vi "CreateDUTNode.vi"(7 "DOM Document":refnum<k20>, 8 "Error In":errorcluster, 11 "DUT Configuration":T1={"Count"=1, "Wirings"=[], "Names"=[]}) -> (0 "Error Out":errorcluster, 3 "DUT Node":refnum<k20>)   [LabVIEW 2013]
uses:
  DUTConfiguration.ctl
  driver/Public/Controls/SMUSense.ctl
  libs/LV-Utilities/LV-Utilities.lvlib
  driver/Keithley-2602.lvlib
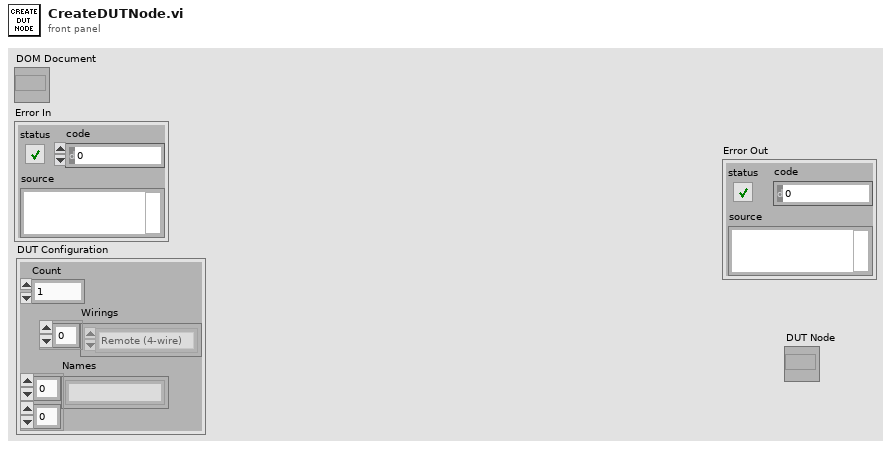
[diagram p1: front panel]
types:
  T1 = typedef "DUTConfiguration.ctl" = cluster{"Count":u32, "Wirings":T2[], "Names":string[][]}
  T2 = typedef "Keithley-2602.lvlib/SMUSense.ctl" = enum16{"Local (2-wire)", "Remote (4-wire)", "Calibration"}
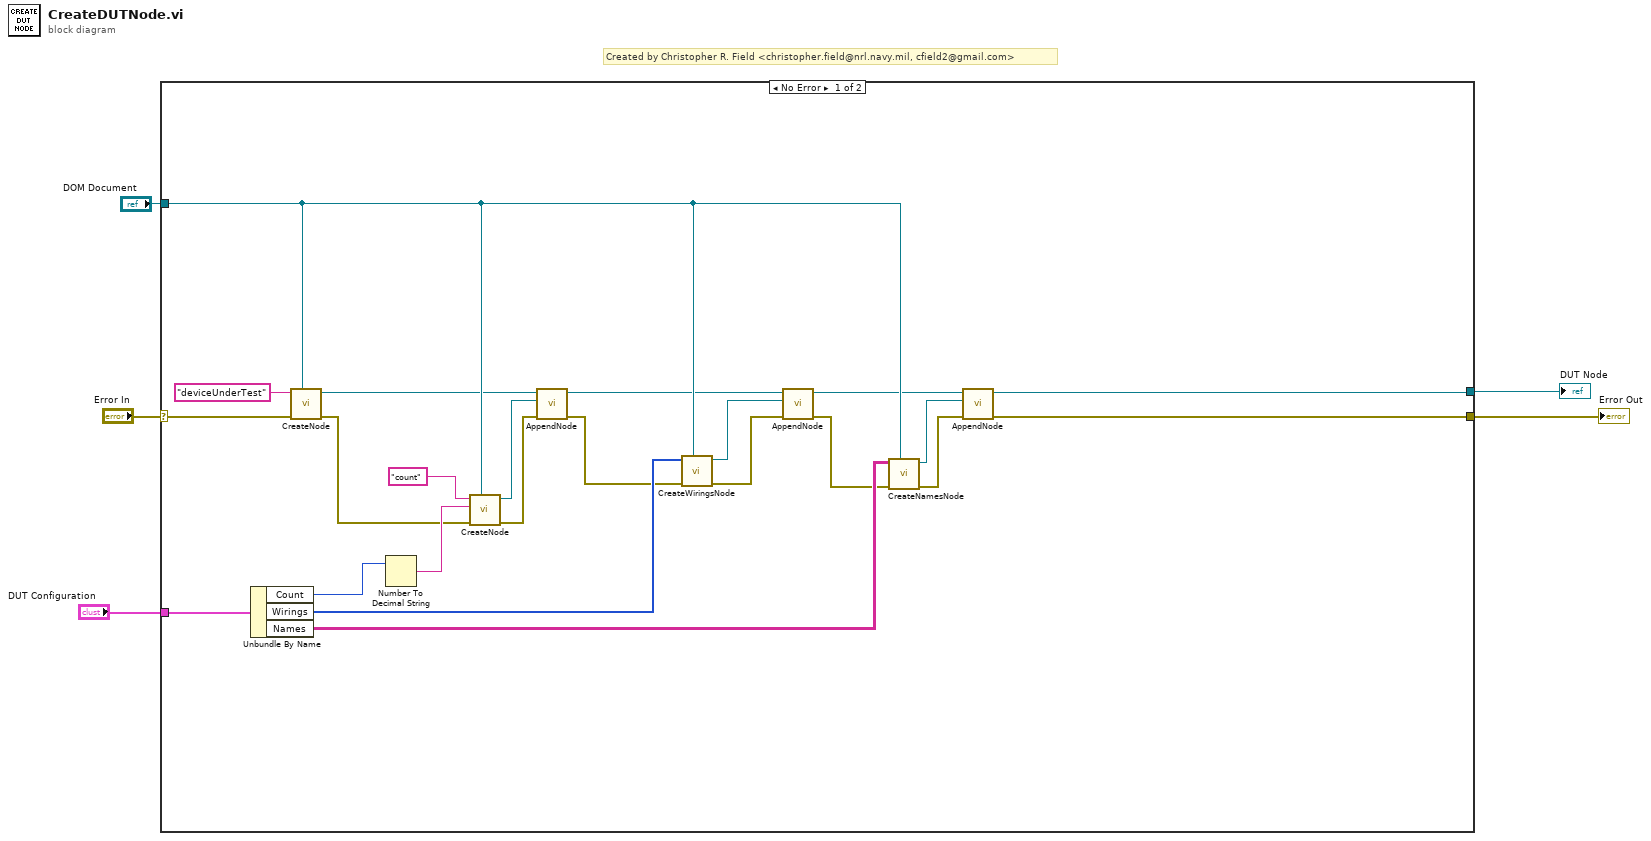
[diagram p0: block diagram]
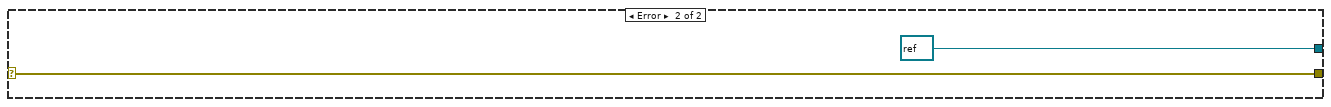
[diagram p2: hidden frame]
diagram:
  # "Created by Christopher R. Field <christopher.field@nrl.navy.mil, cfield2@gmail.com>"
  n1 = case shown="No Error" "Error In" {
    selector: "Error In" -> [w22 w30]
    tunnel: "DOM Document" -> [w20 _]
    tunnel: [w14 w30] -> w3
    tunnel: [w15 refnum<k20> refnum ("DUT Node 2")] -> w2
    tunnel: "DUT Configuration" -> [w23 _]
    frame No Error {
      n2 = Unbundle By Name(w23) -> ("Count"=w28:u32, "Wirings"=w25:T2[], "Names"=w24:string[][])
      n3 = call "CreateNode.vi"("DOM Document"=w20, "Error In"=w22, "Tag Name"="deviceUnderTest") -> ("Error out"=w6:errorcluster, "Node"=w19:refnum<k20>)  [unwired: 7 in]
      n4 = Number To Decimal String(number=w28) -> (decimal integer string=w26:string)  [unwired: 1 in]
      n5 = call "CreateNode.vi"("DOM Document"=w20, "Error In"=w6, "Text"=w26, "Tag Name"="count") -> ("Error out"=w7:errorcluster, "Node"=w18:refnum<k20>)  [unwired: 6 in]
      n6 = call "AppendNode.vi"("Error In"=w7, "Child Node"=w18, "Parent Node In"=w19) -> ("Error Out"=w8:errorcluster, "Parent Node Out"=w17:refnum<k20>)  [unwired: 7 in]
      n7 = call "CreateWiringsNode.vi"("DOM Document"=w20, "Error In"=w8, "Wirings"=w25) -> ("Error Out"=w10:errorcluster, "Wirings Node"=w9:refnum<k20>)  [unwired: 7 in]
      n8 = call "AppendNode.vi"("Error In"=w10, "Child Node"=w9, "Parent Node In"=w17) -> ("Error Out"=w11:errorcluster, "Parent Node Out"=w16:refnum<k20>)  [unwired: 7 in]
      n9 = call "CreateNamesNode.vi"("DOM Document"=w20, "Error In"=w11, "Names"=w24) -> ("Error Out"=w13:errorcluster, "Names Node"=w12:refnum<k20>)  [unwired: 7 in]
      n10 = call "AppendNode.vi"("Error In"=w13, "Child Node"=w12, "Parent Node In"=w16) -> ("Error Out"=w14:errorcluster, "Parent Node Out"=w15:refnum<k20>)  [unwired: 7 in]
    }
    frame Error {
    }
  }
  "Error Out" <- w3
  "DUT Node" <- w2
